vi "SimpleMotorFF_MaxAchieveVel.vi"(9 "Acceleration":dbl, 10 "MaxVoltage":dbl, 11 "SIMPLE_MOTOR_FF":T1 {"KnInv" format="%13.4f"; "Ka" format="%13.4f"; "Kv" format="%13.4f"; "Ks" format="%13.4f"}) -> (3 "MaxVelocity":dbl)   [LabVIEW 2019, in "Trajectory_Library.lvlib"]
doc: "Calculates the maximum achievable velocity given a maximum voltage supply and an acceleration. Useful for ensuring that velocity and acceleration constraints for a trapezoidal profile are simultaneously achievable - enter the acceleration constraint, and this will give you a simultaneously-achievable velocity constraint.\n\nParameters:\n - Simple_Motor_FF - Data structure containing constants\n - maxVoltage -The maximum voltage that can be supplied to the motor.\n - Acceleration - The acceleration of the motor.\n\nReturns:\n MaxVelocity - The maximum possible velocity at the given acceleration."
uses:
  Trajectory_Library.lvlib
  TypeDef/SIMPLE_MOTOR_FF.ctl
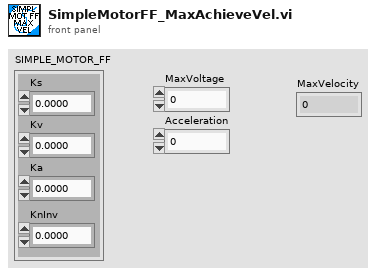
[diagram p1: front panel]
types:
  T1 = typedef "Trajectory_Library.lvlib/SIMPLE_MOTOR_FF.ctl" = cluster{"Ks":dbl, "Kv":dbl, "Ka":dbl, "KnInv":dbl}
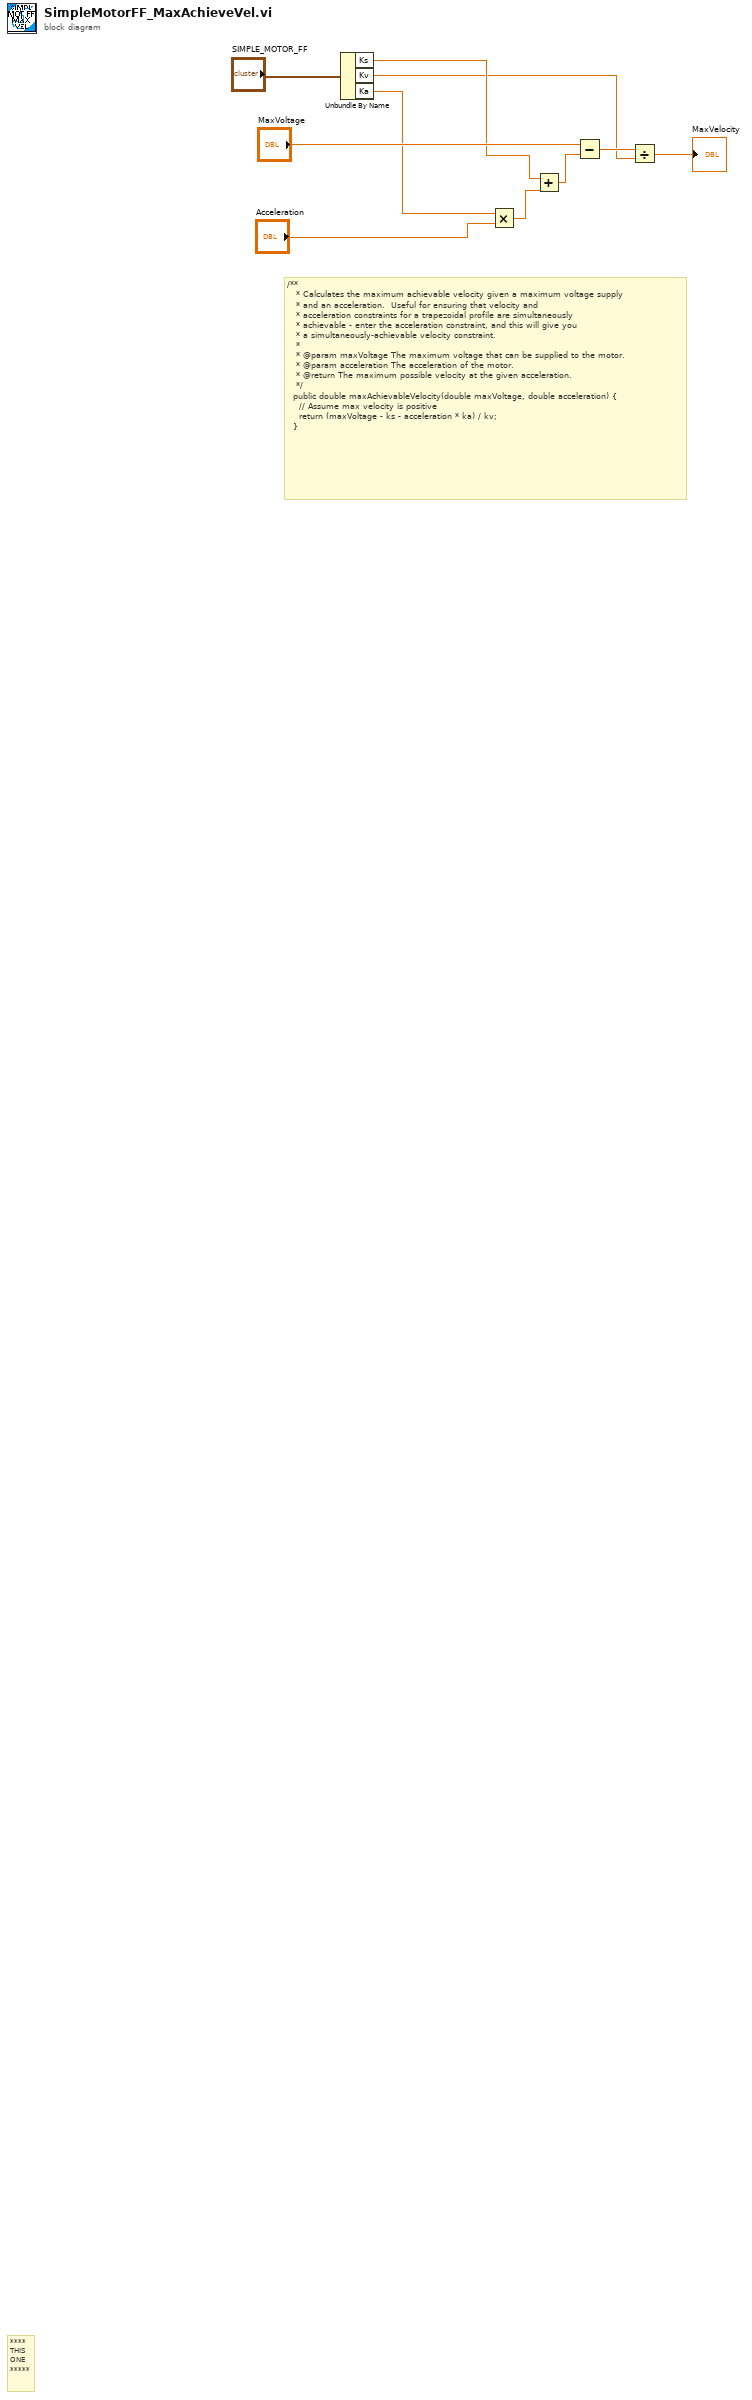
[diagram p0: block diagram]
diagram:
  # "/**\n   * Calculates the maximum achievable velocity given a maximum voltage supply\n   * and an acceleration.  Useful for ensuring that velocity and\n   * acceleration constraints for a trapezoidal profile are simultaneously\n   * achievable - enter the acceleration constraint, and this will give you\n   * a simultaneously-achievable velocity constraint.\n   *\n   * @param maxVoltage The maximum voltage that can be supplied to the motor.\n   * @param acceleration The acceleration of the motor.\n   * @return The maximum possible velocity at the given acceleration.\n   */\n  public double maxAchievableVelocity(double maxVoltage, double acceleration) {\n    // Assume max velocity is positive\n    return (maxVoltage - ks - acceleration * ka) / kv;\n  }"
  # "****\nTHIS\nONE\n*****"
  n1 = Unbundle By Name("SIMPLE_MOTOR_FF") -> ("Ks"=w3:dbl, "Kv"=w1:dbl, "Ka"=w2:dbl)
  n2 = Multiply(x=w2, y="Acceleration") -> (x*y=w7:dbl)
  n3 = Add(x=w3, y=w7) -> (x+y=w6:dbl)
  n4 = Subtract(x="MaxVoltage", y=w6) -> (x-y=w5:dbl)
  n5 = Divide(x=w5, y=w1) -> (x/y=→"MaxVelocity":dbl)
